vi "Query Output Relative Power.vi"(8 "error in (no error)":errorcluster, 9 "Relative Power Type (0:Current)":u16(ring) items=["Current", "MINimum", "MAXimum", "DEFault"], 10 "Platform Slot Number (10)":i16=10 min=-1 max=255, 11 "VISA resource name":refnum<visa-resource-name>) -> (0 "error out":errorcluster, 2 "Relative Power":dbl format="%#_6e", 3 "VISA resource name out":refnum<visa-resource-name>)   [LabVIEW 2018, in "LTB-1.lvlib" / "3150.lvlib"]
doc: "Queries the value indicating the current or the minimum/maximum/default value of relative power value, in dBM.\n\n<B>Note:</B>\nThis command is applicable only for <B>Self-adjusting module</B> type of 3150. For standard module, \"Power control option not available.\" message will be returned as it doesn't support Output Power control mode. Refer IQS-3150 user manual for more information."
uses:
  3150.lvlib
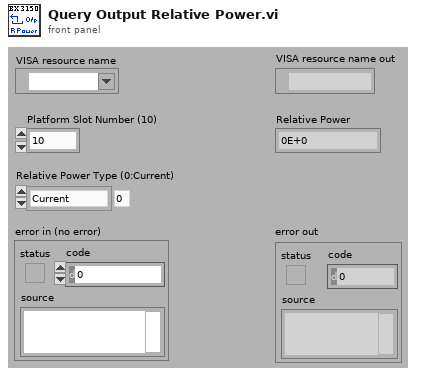
[diagram p1: front panel]
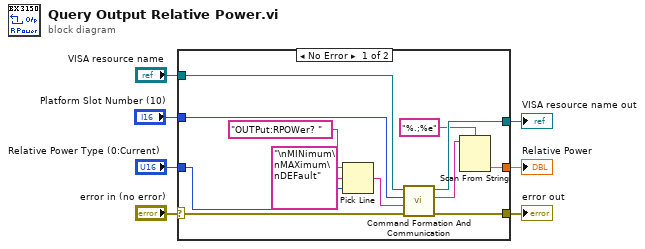
[diagram p0: block diagram]
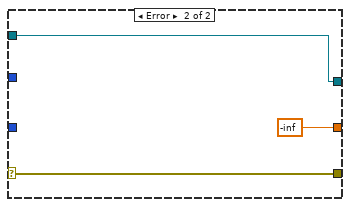
[diagram p2: hidden frame]
diagram:
  n1 = case shown="No Error" "error in (no error)" {
    selector: "error in (no error)" -> [w18 w21]
    tunnel: "VISA resource name" -> [w19 w22]
    tunnel: [w17 w22] -> w5
    tunnel: [w16 w21] -> w4
    tunnel: "Relative Power Type (0:Current)" -> [w14 _]
    tunnel: "Platform Slot Number (10)" -> [w13 _]
    tunnel: [w10 -inf] -> w1
    frame No Error {
      n2 = Pick Line(string ("")="OUTPut:RPOWer? " ("Command"), multi-line string="\nMINimum\nMAXimum\nDEFault" ("input 1"), line index=w14) -> (output string=w8:string)
      n3 = call "Command Formation And Communication.vi"("error in (no error)"=w18, "Command"=w8, "Platform Slot Number"=w13, "VISA resource name"=w19) -> ("error out"=w16:errorcluster, "Response"=w12:string, "VISA resource name out"=w17:refnum<visa-resource-name>)  [unwired: 1 in, 4 out]
      n4 = Scan From String(format string="%.;%e", input string=w12) -> (output 1=w10:dbl)  [unwired: 2 in, 4 out]
    }
    frame Error {
    }
  }
  "VISA resource name out" <- w5
  "error out" <- w4
  "Relative Power" <- w1
